vi "Dispose.vi"(8 "error in (no error)":errorcluster, 11 "Redis Pipelining TCP Client in":refnum<class "Redis Pipelining TCP Client.lvclass">) -> (0 "error out":errorcluster)   [LabVIEW 2019, in "Redis Client for LabVIEW.lvlib" / "Redis Pipelining TCP Client.lvclass"]
uses:
  Redis Pipelining TCP Client.lvclass
  Redis Pipelining TCP Client.lvclass/Redis Pipelining TCP Client.ctl
  Redis TCP Client/Redis TCP Client.lvclass
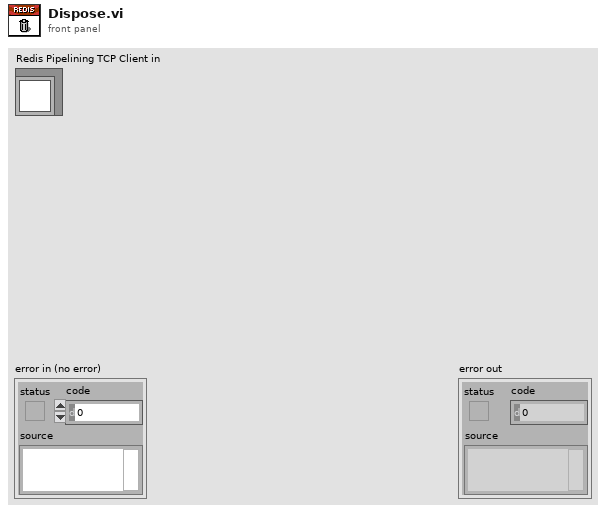
[diagram p1: front panel]
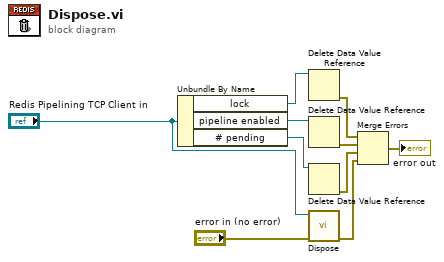
[diagram p0: block diagram]
diagram:
  n1 = Unbundle By Name("Redis Pipelining TCP Client in") -> ("lock"=w2:refnum<data-value>, "pipeline enabled"=w4:refnum<data-value>, "# pending"=w8:refnum<data-value>)
  n2 = Delete Data Value Reference(data value reference=w2) -> (error out=w1:errorcluster)  [unwired: 1 in, 1 out]
  n3 = Delete Data Value Reference(data value reference=w4) -> (error out=w3:errorcluster)  [unwired: 1 in, 1 out]
  n4 = Delete Data Value Reference(data value reference=w8) -> (error out=w7:errorcluster)  [unwired: 1 in, 1 out]
  n5 = call-parent "Dispose.vi"("error in (no error)"="error in (no error)", "Redis TCP Client in"="Redis Pipelining TCP Client in") -> ("error out"=w6:errorcluster)  [unwired: 9 in]
  n6 = Merge Errors(w1, w3, w7, w6) -> (→"error out":errorcluster)
